vi "Create Plugin.vi"(5 "Debug Flags":refnum<class "Debug Flags.lvclass">, 8 "error in (no error)":errorcluster, 9 "component classes":refnum<class>[](array[class]), 10 "Plugin Configuration":T1={"name"="", "class"="", "cycle timing"={"priority"=0, "decimation"=1, "offset"=0}, "Transfer Groups"=[], "settings"=[], "thread count"=0} {"Transfer Groups"."Transfers"."channel configurations"."buffer offset" format="%d bytes"}, 11 "Transfer Groups":refnum<class "Transfer Group.lvclass">[](array[class])) -> (0 "error out":errorcluster, 1 "Buffer Converter":refnum<class "Buffer Converter.lvclass">, 2 "Transceiver":refnum<class "Transceiver.lvclass">, 3 "Plugin out":refnum<class "Plugin.lvclass">)   [LabVIEW 2017, in "DSF Core.lvlib" / "Plugin.lvclass"]
uses:
  Plugin.lvclass
  Transfer Group/Transfer Group.lvclass
  Debug/Debug Flags/Debug Flags.lvclass
  Configuration/Public/Controls/DSF Engine Plugin Configuration.ctl
  Configuration/Public/Controls/DSF Timing Info.ctl
  Configuration/Public/Controls/DSF Engine Transfer Group Configuration.ctl
  Configuration/Public/Controls/DSF Direction.ctl
  Configuration/Public/Controls/DSF Engine Transfer Configuration.ctl
  Configuration/Public/Controls/DSF Byte Order.ctl
  Configuration/Public/Controls/DSF Engine Channel Configuration.ctl
  Configuration/Public/Controls/DSF Data Type.ctl
  Configuration/Public/Controls/DSF Settings Info.ctl
  Transceiver/Transceiver.lvclass
  Buffer Converter/Buffer Converter.lvclass
  Plugin.lvclass/Plugin.ctl
  Timing/Timing.lvclass
  DSF Core.lvlib
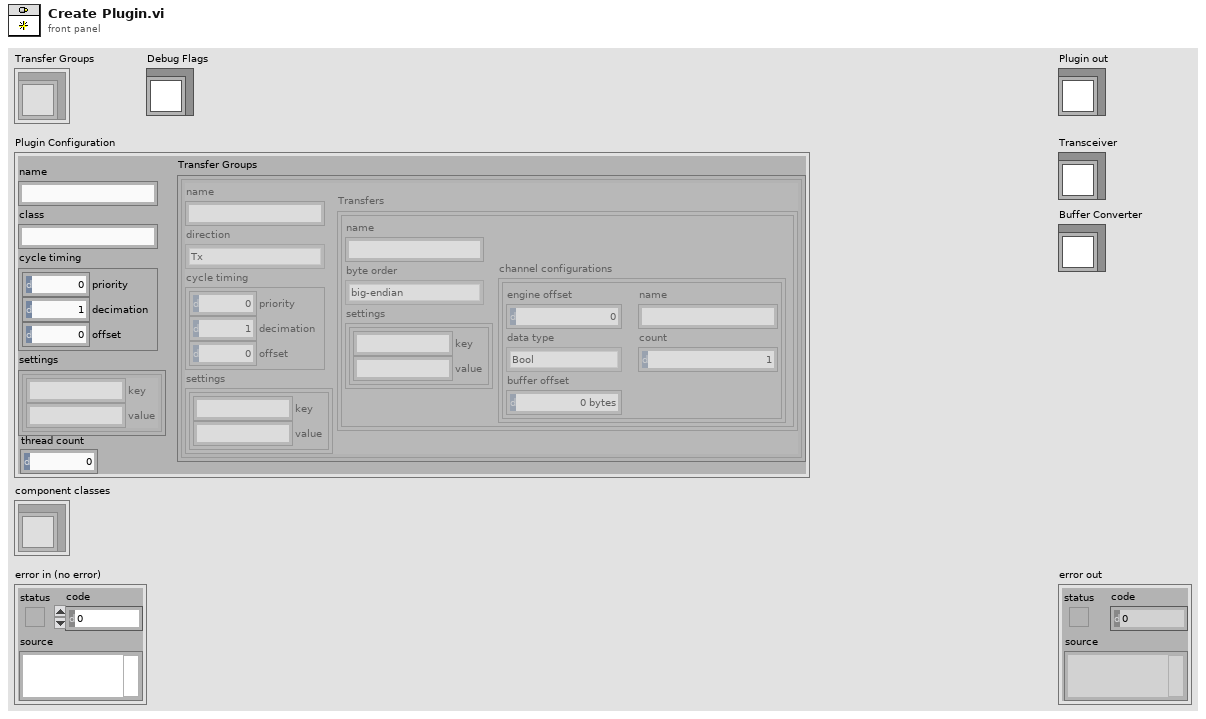
[diagram p1: front panel]
types:
  T1 = typedef "DSF Core.lvlib/DSF Engine Plugin Configuration.ctl" = cluster{"name":string, "class":string, "cycle timing":T2, "Transfer Groups":T3[], "settings":T9, "thread count":i32}
  T2 = typedef "DSF Core.lvlib/DSF Timing Info.ctl" = cluster{"priority":u64, "decimation":u64, "offset":u64}
  T3 = typedef "DSF Core.lvlib/DSF Engine Transfer Group Configuration.ctl" = cluster{"name":string, "direction":T4, "cycle timing":T2, "Transfers":T5[], "settings":T9}
  T4 = typedef "DSF Core.lvlib/DSF Direction.ctl" = enum8{"Tx", "Rx"}
  T5 = typedef "DSF Core.lvlib/DSF Engine Transfer Configuration.ctl" = cluster{"name":string, "byte order":T6, "channel configurations":T7[], "settings":T9}
  T6 = typedef "DSF Core.lvlib/DSF Byte Order.ctl" = enum8{"big-endian", "little-endian"}
  T7 = typedef "DSF Core.lvlib/DSF Engine Channel Configuration.ctl" = cluster{"engine offset":u64, "name":string, "data type":T8, "count":u64, "buffer offset":u64}
  T8 = typedef "DSF Core.lvlib/DSF Data Type.ctl" = enum8{"Bool", "SGL", "DBL", "I8", "I16", "I32", "I64", "U8", "U16", "U32", "U64"}
  T9 = typedef "DSF Core.lvlib/DSF Settings Info.ctl" = cluster{"key":string, "value":string}[]
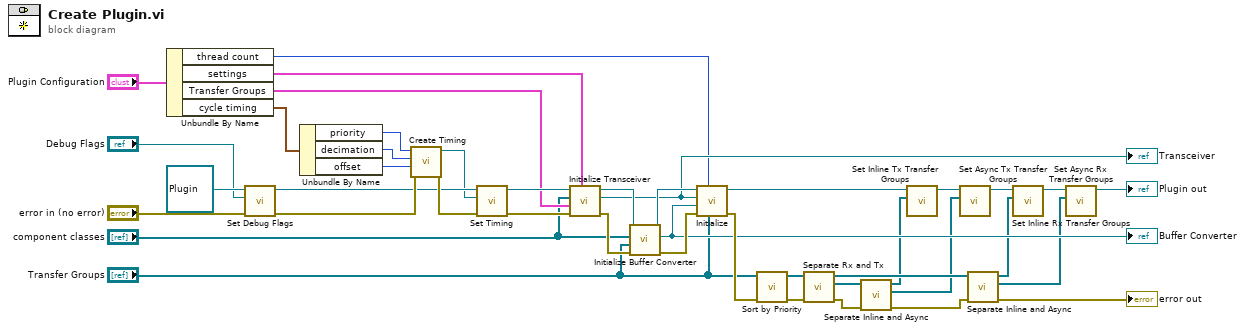
[diagram p0: block diagram]
diagram:
  n1 = Unbundle By Name("Plugin Configuration") -> ("thread count"=w9:i32, "settings"=w10:T9, "Transfer Groups"=w21:T3[], "cycle timing"=w11:T2)
  n2 = call "Set Debug Flags.vi"("Debug Flags"="Debug Flags", "Plugin in"=refnum<class "Plugin.lvclass"> refnum) -> ("Plugin out"=w7:refnum<class "Plugin.lvclass">)  [unwired: 9 in]
  n3 = Unbundle By Name(w11) -> ("priority"=w22:u64, "decimation"=w23:u64, "offset"=w24:u64)
  n4 = call "Create Timing.vi"("error in (no error)"="error in (no error)", "Offset"=w24, "Decimation"=w23, "Priority"=w22) -> ("error out"=w38:errorcluster, "Timing"=w5:refnum<class "Timing.lvclass">)  [unwired: 6 in]
  n5 = call "Set Timing.vi"("Timing"=w5, "Plugin in"=w7) -> ("Plugin out"=w40:refnum<class "Plugin.lvclass">)  [unwired: 9 in]
  n6 = call "Initialize Transceiver.vi"("transceiver settings"=w10, "error in (no error)"=w38, "Transfer Groups Configurations"=w21, "component classes"="component classes", "Plugin in"=w40) -> ("error out"=w20:errorcluster, "Transceiver"=w16:refnum<class "Transceiver.lvclass">, "Plugin out"=w18:refnum<class "Plugin.lvclass">)  [unwired: 4 in]
  "Transceiver" <- w16
  n7 = call "Initialize Buffer Converter.vi"("error in (no error)"=w20, "Transfer Groups"="Transfer Groups", "component classes"="component classes", "Plugin in"=w18) -> ("error out"=w19:errorcluster, "Buffer Converter"=w15:refnum<class "Buffer Converter.lvclass">, "Plugin out"=w17:refnum<class "Plugin.lvclass">)  [unwired: 5 in]
  "Buffer Converter" <- w15
  n8 = call "Initialize.vi"("Transfer Groups"="Transfer Groups", "thread count"=w9, "error in (no error)"=w19, "Buffer Converter"=w15, "Transceiver"=w16, "Plugin in"=w17) -> ("error out"=w26:errorcluster, "Plugin out"=w28:refnum<class "Plugin.lvclass">)  [unwired: 4 in]
  n9 = call "Sort by Priority.vi"("error in (no error)"=w26, "Transfer Groups"="Transfer Groups") -> ("error out"=w37:errorcluster, "sorted Transfer Groups"=w36:refnum<class "Transfer Group.lvclass">[])  [unwired: 8 in]
  n10 = call "Separate Rx and Tx.vi"("error in (no error)"=w37, "Transfer Groups"=w36) -> ("error out"=w35:errorcluster, "Tx Transfer Groups"=w34:refnum<class "Transfer Group.lvclass">[], "Rx Transfer Groups"=w33:refnum<class "Transfer Group.lvclass">[])  [unwired: 7 in]
  n11 = call "Separate Inline and Async.vi"("error in (no error)"=w35, "Transfer Groups"=w34) -> ("error out"=w32:errorcluster, "Async Transfer Groups"=w3:refnum<class "Transfer Group.lvclass">[], "Inline Transfer Groups"=w4:refnum<class "Transfer Group.lvclass">[])  [unwired: 7 in]
  n12 = call "Set Inline Tx Transfer Groups.vi"("Inline Tx Transfer Groups"=w4, "Plugin in"=w28) -> ("Plugin out"=w31:refnum<class "Plugin.lvclass">)  [unwired: 9 in]
  n13 = call "Set Async Tx Transfer Groups.vi"("Async Tx Transfer Groups"=w3, "Plugin in"=w31) -> ("Plugin out"=w30:refnum<class "Plugin.lvclass">)  [unwired: 9 in]
  n14 = call "Separate Inline and Async.vi"("error in (no error)"=w32, "Transfer Groups"=w33) -> ("error out"=→"error out":errorcluster, "Async Transfer Groups"=w1:refnum<class "Transfer Group.lvclass">[], "Inline Transfer Groups"=w2:refnum<class "Transfer Group.lvclass">[])  [unwired: 7 in]
  n15 = call "Set Inline Rx Transfer Groups.vi"("Inline Rx Transfer Groups"=w2, "Plugin in"=w30) -> ("Plugin out"=w29:refnum<class "Plugin.lvclass">)  [unwired: 9 in]
  n16 = call "Set Async Rx Transfer Groups.vi"("Async Rx Transfer Groups"=w1, "Plugin in"=w29) -> ("Plugin out"=→"Plugin out":refnum<class "Plugin.lvclass">)  [unwired: 9 in]
